vi "0926New Project.vi"() -> ()   [LabVIEW 2011] (continued)
                          }
                          frame #3 {
                            n542 = local read "Spec_midVar"() -> (w635:string)
                            n543 = property on="Cable AWG:" class="Ring (严格)"() -> ("StringsAndValues[]"=w648:T9)  [unwired: 2 in, 2 out]
                            n544 = property on="Customer" class="Ring (严格)"() -> ("StringsAndValues[]"=w650:T9)  [unwired: 2 in, 2 out]
                            n545 = Search and Replace String(replace all?=TRUE ("替换全部？(F)"), input string=w635, search string="#" ("搜索字符串"), replace string="\t") -> (result string=w639:string)  [unwired: 4 in, 3 out]
                            n546 = local read "Customer"() -> (w649:string)
                            n547 = local read "AWG"() -> (w647:string)
                            n548 = Spreadsheet String To Array(format string="%s" ("格式字符串"), spreadsheet string=w639, array type (2D Dbl)=string[][] []) -> (array=w642:string[][])  [unwired: 1 in]
                            n549 = call "_wmg_downlistValue.vi"(1:"Customer"=w647, 2:"Customer"=w648) -> ("Customer"=w651:u16)
                            n550 = call "_wmg_downlistValue.vi"(1:"Customer"=w649, 2:"Customer"=w650) -> ("Customer"=w652:u16)
                            n551 = Fract/Exp String To Number(string=w642) -> (number=w645:dbl[][])  [unwired: 3 in, 1 out]
                            n552 = local write "Cable AWG:"(w651) -> ()
                            n553 = local write "Customer"(w652) -> ()
                            n554 = local write "Spec _Data"(w645) -> ()
                            n555 = Array To Spreadsheet String(delimiter (Tab)="#" ("分隔符(Tab)"), array=w645, 3:"%s" ("格式字符串")) -> (spreadsheet string=w646:string)
                            n556 = local write "Spec String"(w646) -> ()
                          }
                        }
                      }
                    }
                  }
                  frame #1 {
                    # "列数\n0. S-para Pair Name\n1. NEXT Pair Name\n2. FEXT Pair Name\n3. Diff TestItems\n4. Single TestItems\n5. TDR TestItems\n6. Spec Associate\n7. VNA Cal File Path\n8. Report Config\n9. ILD Spec\n10. TDR Setting"
                    # "解析Prjinf"
                    n557 = local read "Project Information"() -> (w681:string)
                    n558 = Spreadsheet String To Array(delimiter (Tab)="#" ("分隔符(Tab)"), format string="%s" ("格式字符串"), spreadsheet string=w681, array type (2D Dbl)=string[][] []) -> (array=w678:string[][])
                    n559 = Index Array(array=w678, index (col) #1=0 ("索引"), index (col) #2=1 ("索引 (列)"), index (col) #3=2 ("索引 (列)"), index (col) #4=3 ("索引 (列)"), index (col) #5=4 ("索引 (列)"), index (col) #6=5 ("索引"), index (col) #7=6 ("索引 (列)"), index (col) #8=7 ("索引 (列)"), index (col) #9=8 ("索引 (列)"), index (col) #10=9 ("索引 (列)"), index (col) #11=10 ("索引"), index (col) #12=11 ("索引 (列)")) -> (element #1=w677:string[], element #2=w676:string[], element #3=w675:string[], element #4=w674:string[], element #5=w673:string[], element #6=w672:string[], element #7=w671:string[], element #8=w670:string[], element #9=w669:string[], element #10=w668:string[], element #11=w667:string[], element #12=w653:string[])  [unwired: 12 in]
                    n560 = stacked-sequence {
                      tunnel: w677 -> [_ w693 _ _ _]
                      tunnel: w676 -> [_ w692 _ _ _]
                      tunnel: w675 -> [_ w691 _ _ _]
                      tunnel: w674 -> [_ w690 _ _ _]
                      tunnel: w673 -> [_ w689 _ _ _]
                      tunnel: w672 -> [_ w688 _ _ _]
                      tunnel: w671 -> [_ _ w744 _ _]
                      tunnel: w670 -> [_ _ w743 _ _]
                      tunnel: w669 -> [_ _ _ w767 _]
                      tunnel: w668 -> [_ _ _ _ _]
                      tunnel: w667 -> [_ _ _ _ w785]
                      tunnel: w653 -> [_ _ w740 _ _]
                      frame #0 {
                        n561 = local read "Single init"() -> (→"Single init 2":i32[])
                        n562 = local read "NEXT init"() -> (→"NEXT init 2":i32[])
                        n563 = local read "FEXT init"() -> (→"FEXT init 2":i32[])
                        n564 = local read "S-p init"() -> (→"S-p init 2":i32[])
                        n565 = local read "Diff init"() -> (→"Diff init 2":i32[])
                        n566 = local read "TDR init"() -> (→"TDR init 2":i32[])
                      }
                      frame #1 {
                        n567 = stacked-sequence {
                          tunnel: [_ w715 _ _] -> _
                          tunnel: w693 -> [_ w715 _ _]
                          tunnel: w692 -> [_ w708 _ _]
                          tunnel: w691 -> [_ _ w721 _]
                          tunnel: w690 -> [_ _ w716 _]
                          tunnel: w689 -> [_ _ _ w729]
                          tunnel: w688 -> [_ _ _ w726]
                          frame #0 {
                            n568 = local read "FEXT init"() -> (w701:string[])
                            n569 = local read "FEXT init"() -> (w700:i32[])
                            n570 = local read "NEXT init"() -> (w704:string[])
                            n571 = local read "NEXT init"() -> (w702:i32[])
                            n572 = local read "S-p init"() -> (w703:i32[])
                            n573 = local read "S-p init"() -> (w705:string[])
                            n574 = property on="S-para Pair Name" class="LstBox (严格)"("Item Names"=w705, "Item Symbols"=w703) -> ()  [unwired: 2 in, 2 out]
                            n575 = property on="NEXT Pair Name" class="LstBox (严格)"("Item Names"=w704, "Item Symbols"=w702) -> ()  [unwired: 2 in, 2 out]
                            n576 = property on="FEXT Pair Name" class="LstBox (严格)"("Item Names"=w701, "Item Symbols"=w700) -> ()  [unwired: 2 in, 2 out]
                            n577 = local read "Single init"() -> (w697:string[])
                            n578 = local read "Single init"() -> (w696:i32[])
                            n579 = local read "TDR init"() -> (w695:string[])
                            n580 = local read "TDR init"() -> (w694:i32[])
                            n581 = local read "Diff init"() -> (w699:string[])
                            n582 = local read "Diff init"() -> (w698:i32[])
                            n583 = property on="Diff Test Items" class="LstBox (严格)"("Item Names"=w699, "Item Symbols"=w698) -> ()  [unwired: 2 in, 2 out]
                            n584 = property on="Single Test Items" class="LstBox (严格)"("Item Names"=w697, "Item Symbols"=w696) -> ()  [unwired: 2 in, 2 out]
                            n585 = property on="TDR Test Items" class="LstBox (严格)"("Item Names"=w695, "Item Symbols"=w694) -> ()  [unwired: 2 in, 2 out]
                          }
                          frame #1 {
                            n586 = local read "S-p init"() -> (w713:i32[])
                            n587 = local read "NEXT init"() -> (w706:string[])
                            n588 = local read "NEXT init"() -> (w709:i32[])
                            n589 = local read "S-p init"() -> (w707:string[])
                            n590 = call "_wmg_readItems.vi"("input_p"=w713, "input"=w707, "input_sp"=w715) -> ("output_p"=w712:i32[], "output_sp"=w714:string[])
                            n591 = call "_wmg_readItems2.vi"("input_p"=w709, "input"=w706, "input_sp"=w708) -> ("output_p"=w710:i32[], "output_sp"=w711:string[])
                            n592 = property on="S-para Pair Name" class="LstBox (严格)"("Item Names"=w714, "Item Symbols"=w712) -> ()  [unwired: 2 in, 2 out]
                            n593 = property on="NEXT Pair Name" class="LstBox (严格)"("Item Names"=w711, "Item Symbols"=w710) -> ()  [unwired: 2 in, 2 out]
                          }
                          frame #2 {
                            n594 = local read "FEXT init"() -> (w724:string[])
                            n595 = local read "FEXT init"() -> (w725:i32[])
                            n596 = local read "Diff init"() -> (w720:string[])
                            n597 = local read "Diff init"() -> (w719:i32[])
                            n598 = call "_wmg_readItems2.vi"("input_p"=w719, "input"=w720, "input_sp"=w716) -> ("output_p"=w718:i32[], "output_sp"=w717:string[])
                            n599 = call "_wmg_readItems.vi"("input_p"=w725, "input"=w724, "input_sp"=w721) -> ("output_p"=w722:i32[], "output_sp"=w723:string[])
                            n600 = property on="FEXT Pair Name" class="LstBox (严格)"("Item Names"=w723, "Item Symbols"=w722) -> ()  [unwired: 2 in, 2 out]
                            n601 = property on="Diff Test Items" class="LstBox (严格)"("Item Names"=w717, "Item Symbols"=w718) -> ()  [unwired: 2 in, 2 out]
                          }
                          frame #3 {
                            n602 = local read "TDR init"() -> (w728:string[])
                            n603 = local read "TDR init"() -> (w727:i32[])
                            n604 = local read "Single init"() -> (w730:string[])
                            n605 = local read "Single init"() -> (w731:i32[])
                            n606 = call "_wmg_readItems.vi"("input_p"=w731, "input"=w730, "input_sp"=w729) -> ("output_p"=w733:i32[], "output_sp"=w732:string[])
                            n607 = call "_wmg_readItems2.vi"("input_p"=w727, "input"=w728, "input_sp"=w726) -> ("output_p"=w735:i32[], "output_sp"=w734:string[])
                            n608 = property on="TDR Test Items" class="LstBox (严格)"("Item Names"=w734, "Item Symbols"=w735) -> ()  [unwired: 2 in, 2 out]
                            n609 = property on="Single Test Items" class="LstBox (严格)"("Item Names"=w732, "Item Symbols"=w733) -> ()  [unwired: 2 in, 2 out]
                          }
                        }
                      }
                      frame #2 {
                        n610 = property on="Diff Test Items" class="LstBox (严格)"() -> ("Item Symbols"=w749:i32[], "Item Names"=w747:string[])  [unwired: 2 in, 2 out]
                        n611 = Index Array(array=w743, index=0 ("索引")) -> (element=w742:string)
                        n612 = Index Array(array=w740, index=0 ("索引")) -> (element=w738:string)
                        n613 = local write "VNA Cal File Path:"(w742) -> ()
                        n614 = Equal?(x=w738, y="TRUE") -> (x = y?=w736:bool)
                        n615 = for {
                          tunnel: w749 -> [w755] mode=indexing
                          shift-right: [w750] -> w746
                          shift-left: string[] [] -> [w751]
                          tunnel: w747 -> [w752] mode=indexing
                          n616 = Equal?(x=w755, y=38) -> (x = y?=w753:bool)
                          n617 = case shown="假" w753 {
                            tunnel: w752 -> [_ w759]
                            tunnel: w751 -> [w756 w758]
                            tunnel: [w756 w757] -> w750
                            frame False {
                            }
                            frame True {
                              n618 = Insert Into Array(array=w758, new element=w759) -> (w757:string[])  [unwired: 1 in]
                            }
                          }
                        }
                        n619 = local write "cancel dem2X?"(w736) -> ()
                        n620 = Build Array(w746, w744) -> (w745:string[][])
                        n621 = local write "Spec Associate"(w745) -> ()
                      }
                      frame #3 {
                        n622 = Index Array(array=w767, index #1=0 ("索引"), index #3=2 ("索引")) -> (element #1=w764:string, element #2=w763:string, element #3=w761:string)  [unwired: 1 in]
                        n623 = String To Path(string=w764) -> (path=w765:path)
                        n624 = call "_wmg_ReportConfigDivided@.vi"("Input"=w763) -> ("Output"=w762:string[][])
                        n625 = call "_wmg_ReportConfigDivided@.vi"("Input"=w761) -> ("Output"=w760:string[][])
                        n626 = local write "Postion for Raw data"(w762) -> ()
                        n627 = local write "Report Templete Path:"(w765) -> ()
                        n628 = local write "Postion for \"PN&Tester&Date\" etc Fields"(w760) -> ()
                      }
                      frame #4 {
                        # "TDR Setting\n0. Start TimeNs\n1. Stop TimeNs\n2. Data Points\n3. Filter Risetime(ps)\n4. Compensation(ohm)\n5. Impedance Filter\n6. Impedance Spec:\n7. Delay Spec:\n8. skew Spec:\n9. IL 2X Data:"
                        n629 = Index Array(array=w785, index #1=0 ("索引"), index #2=1 ("索引"), index #3=2 ("索引"), index #4=3 ("索引"), index #5=4 ("索引"), index #6=5 ("索引"), index #7=6 ("索引"), index #8=9 ("索引")) -> (element #1=w777:string, element #2=w776:string, element #3=w775:string, element #4=w774:string, element #5=w773:string, element #6=w772:string, element #7=w771:string, element #8=w769:string)
                        n630 = stacked-sequence {
                          tunnel: w777 -> [w810]
                          tunnel: w776 -> [w807]
                          tunnel: w775 -> [w805]
                          tunnel: w774 -> [w804]
                          tunnel: w773 -> [w801]
                          tunnel: w772 -> [w799]
                          tunnel: w771 -> [w796]
                          tunnel: w769 -> [w791]
                          frame #0 {
                            n631 = call "_wmg_ImpSpecDivided@.vi"("Input"=w796) -> ("Output"=w795:string[][])
                            n632 = Spreadsheet String To Array(format string="%s" ("格式字符串"), spreadsheet string=w791, array type (2D Dbl)=dbl[] []) -> (array=w786:dbl[])  [unwired: 1 in]
                            n633 = Insert Into Array(array=w795, index (col)=0 ("禁用的索引 (列)"), new element=string[] ["Mating Area", "Cable Area"]) -> (w793:string[][])  [unwired: 1 in]
                            n634 = local write "2X Thru  IL Data"(w786) -> ()
                            n635 = Decimal String To Number(string=w799) -> (offset past number=w800:i32)  [unwired: 2 in, 1 out]
                            n636 = local write "Impedance Spec:"(w793) -> ()
                            n637 = Number To Boolean Array(number=w800) -> (Boolean array=w798:bool[])
                            n638 = Array To Spreadsheet String(array=w786, 3:"%s" ("格式字符串")) -> (spreadsheet string=w788:string)  [unwired: 1 in]
                            n639 = Fract/Exp String To Number(string=w801) -> (number=w802:dbl)  [unwired: 3 in, 1 out]
                            n640 = Index Array(array=w798) -> (element=w797:bool)  [unwired: 1 in]
                            n641 = Fract/Exp String To Number(string=w807) -> (number=w808:dbl)  [unwired: 3 in, 1 out]
                            n642 = Decimal String To Number(string=w805) -> (number=w806:i32)  [unwired: 2 in, 1 out]
                            n643 = Fract/Exp String To Number(string=w804) -> (number=w803:dbl)  [unwired: 3 in, 1 out]
                            n644 = local write "2X Thru String"(w788) -> ()
                            n645 = local write "Compensation(ohm)"(w802) -> ()
                            n646 = Fract/Exp String To Number(string=w810) -> (number=w809:dbl)  [unwired: 3 in, 1 out]
                            n647 = local write "Filter Risetime(ps)"(w803) -> ()
                            n648 = local write "Impedance Filter"(w797) -> ()
                            n649 = local write "Start TimeNs"(w809) -> ()
                            n650 = local write "StopTimeNs"(w808) -> ()
                            n651 = local write "Data Points"(w806) -> ()
                          }
                        }
                      }
                    }
                  }
                  frame #2 {
                    w819 = T3 {"Row"=0, "Column"=0} ("编辑位置")
                    w820 = u32 4 ("列数")
                    n652 = property on="Single Test Items" class="LstBox (严格)"() -> ("Item Names"=w827:string[], "Item Symbols"=w826:i32[])  [unwired: 2 in, 2 out]
                    n653 = property on="TDR Test Items" class="LstBox (严格)"() -> ("Item Names"=w825:string[], "Item Symbols"=w824:i32[])  [unwired: 2 in, 2 out]
                    n654 = property on="Diff Test Items" class="LstBox (严格)"() -> ("Item Names"=w829:string[], "Item Symbols"=w828:i32[])  [unwired: 2 in, 2 out]
                    n655 = call "_wmg_SelectItems2.vi"("Item Syms"=w824, "Item name"=w825) -> ("Selected tem"=w823:string[])  [unwired: 7 in, 2 out]
                    n656 = call "_wmg_SelectItems2.vi"("Item Syms"=w828, "Item name"=w829) -> ("Selected tem"=w822:string[])  [unwired: 7 in, 2 out]
                    n657 = call "_wmg_SelectItems2.vi"("Item Syms"=w826, "Item name"=w827) -> ("Selected tem"=w821:string[])  [unwired: 7 in, 2 out]
                    n658 = property on="Postion for Raw data" class="Tbl (严格)"() -> ("Value"=w818:string[][])  [unwired: 2 in, 2 out]
                    n659 = Insert Into Array(array=w823, new element #1=w822, new element #2=w821) -> (w817:string[])  [unwired: 1 in]
                    n660 = local read "2X Thru  IL Data"() -> (w813:dbl[])
                    n661 = Replace Array Subset(array=w818, new element=w817, index (col)=0 ("禁用的索引 (列)")) -> (w816:string[][])  [unwired: 1 in]
                    n662 = property on="Postion for Raw data" class="Tbl (严格)"("Value"=w816) -> ()  [unwired: 2 in, 2 out]
                    n663 = Array Size(array=w813) -> (size(s)=w812:i32)
                    n664 = for {
                      N: w812 -> [_]
                      tunnel: [w830] -> w811 mode=indexing
                      i -> [w830]
                    }
                    n665 = Bundle(w811, "2X Thru  IL Data"=w813) -> (w814:cluster{i32[], "2X Thru  IL Data":dbl[]})  [unwired: 1 in]
                    n666 = local write "Insertion Loss"(w814) -> ()
                    n667 = property on="Postion for Raw data" class="Tbl (严格)"("Number of Columns"=w820, "EditPos"=w819) -> ()  [unwired: 2 in, 2 out]
                    n668 = property on="Postion for \"PN&Tester&Date\" etc Fields" class="Tbl (严格)"("Number of Columns"=w820, "EditPos"=w819) -> ()  [unwired: 2 in, 2 out]
                  }
                  frame #3 {
                    n669 = local read "Local"() -> (w831:bool)
                    n670 = case shown="真" w831 {
                      frame False {
                        n671 = local read "result_query"() -> (w835:string)
                        n672 = call <vilib>:"Trim Whitespace.vi"("string"=w835) -> ("trimmed string"=w834:string)  [unwired: 1 in]
                        n673 = String Length(string=w834) -> (length=w833:i32)
                        n674 = Equal To 0?(x=w833) -> (x = 0?=w832:bool)
                        n675 = case shown="假" w832 {
                          frame False {
                            n676 = property on="Update" class="Bool (严格)"("DisabledEnum"=T4."Enabled" ("禁用")) -> ()  [unwired: 2 in, 2 out]
                            n677 = property on="Delete" class="Bool (严格)"("DisabledEnum"=T4."Enabled" ("禁用")) -> ()  [unwired: 2 in, 2 out]
                          }
                          frame True {
                            n678 = local write "Luxshare_P/N:"("") -> ()
                            n679 = One Button Dialog(message="数据库中无此记录" ("消息")) -> ()  [unwired: 1 in, 1 out]
                          }
                        }
                      }
                      frame True {
                        n680 = local read "fileexist"() -> (w841:bool)
                        n681 = Not(x=w841) -> (.not. x?=w840:bool)
                        n682 = case shown="真" w840 {
                          frame False {
                            # "文件不存在"
                            n683 = local read "Impedance Spec:"() -> (w845:string[][])
                            n684 = local write "Luxshare_P/N:"("") -> ()
                            n685 = Replace Array Subset(array=w845, new element=string[] ["", "", ""] ("新元素/子数组"), index (col)=0 ("禁用的索引 (列)")) -> (w844:string[][])  [unwired: 1 in]
                            n686 = local write "Impedance Spec:"(w844) -> ()
                            n687 = property on="Update" class="Bool (严格)"("DisabledEnum"=T4."Disabled and Grayed Out" ("禁用")) -> ()  [unwired: 2 in, 2 out]
                            n688 = property on="Delete" class="Bool (严格)"("DisabledEnum"=T4."Disabled and Grayed Out" ("禁用")) -> ()  [unwired: 2 in, 2 out]
                          }
                          frame True {
                            n689 = property on="Update" class="Bool (严格)"("DisabledEnum"=T4."Enabled" ("禁用")) -> ()  [unwired: 2 in, 2 out]
                            n690 = property on="Delete" class="Bool (严格)"("DisabledEnum"=T4."Enabled" ("禁用")) -> ()  [unwired: 2 in, 2 out]
                          }
                        }
                      }
                    }
                  }
                }
              }
              frame 100 {
                n691 = stacked-sequence {
                  frame #0 {
                    n692 = local read "Local"() -> (w851:bool)
                    n693 = case shown="假" w851 {
                      frame False {
                        n694 = property on="System_Mode" class="Ring (严格)"() -> ("RingText.Text"=w854:string)  [unwired: 2 in, 2 out]
                        n695 = local read "Luxshare_P/N:"() -> (w856:string)
                        n696 = call "_wmg_HardModetoHardModewhereConnect.vi"("Input"=w854) -> ("Output"=w855:string)
                        n697 = call "_wmg_PNtoPNwhereConnect.vi"("Input"=w856) -> ("Output"=w853:string)
                        n698 = Concatenate Strings(w853, w855) -> (w852:string)
                        n699 = call "sql-delete.vi"("操作模式"=T8."删除数据", "限定条件"=w852) -> ()  [unwired: 16 in, 2 out]
                      }
                      frame True {
                        n700 = local read "Luxshare_P/N:"() -> (w859:string)
                        n701 = call <vilib>:"Application Directory.vi"() -> ("Application Directory"=w863:path)
                        n702 = Concatenate Strings("Database\\" ("字符串"), w859, ".hpj" ("字符串")) -> (w862:string)
                        n703 = Build Path(base path=w863, name or relative path=w862) -> (appended path=w858:path)
                        n704 = Delete(path (use dialog)=w858) -> ()  [unwired: 4 in, 3 out]
                      }
                    }
                  }
                  frame #1 {
                    n705 = stacked-sequence {
                      frame #0 {
                        w878 = "@"
                        w879 = "\r\n"
                        w888 = "%s" ("格式字符串")
                        n706 = local read "Impedance Filter"() -> (w865:bool)
                        n707 = local read "Impedance Spec:"() -> (w890:string[][])
                        n708 = local read "2X Thru String"() -> (w875:string)
                        n709 = property on="Skew max(ps)" class="DigNum (严格)"() -> ("NumText.Text"=w867:string)  [unwired: 2 in, 2 out]
                        n710 = property on="Delay(ns)" class="DigNum (严格)"() -> ("NumText.Text"=w874:string)  [unwired: 2 in, 2 out]
                        n711 = property on="Start TimeNs" class="DigNum (严格)"() -> ("NumText.Text"=w873:string)  [unwired: 2 in, 2 out]
                        n712 = property on="StopTimeNs" class="DigNum (严格)"() -> ("NumText.Text"=w872:string)  [unwired: 2 in, 2 out]
                        n713 = property on="Data Points" class="DigNum (严格)"() -> ("NumText.Text"=w871:string)  [unwired: 2 in, 2 out]
                        n714 = property on="Filter Risetime(ps)" class="DigNum (严格)"() -> ("NumText.Text"=w870:string)  [unwired: 2 in, 2 out]
                        n715 = property on="Compensation(ohm)" class="DigNum (严格)"() -> ("NumText.Text"=w869:string)  [unwired: 2 in, 2 out]
                        n716 = Boolean To (0,1)(Boolean=w865) -> (0, 1=w892:i16)
                        n717 = Number To Decimal String(number=w892) -> (decimal integer string=w891:string)  [unwired: 1 in]
                        n718 = call "impedance spec.vi"("Impedance Spec:"=w890) -> ("Impedance spec string"=w889:string)  [unwired: 10 in]
                        n719 = call <vilib>:"Trim Whitespace.vi"("string"=w875) -> ("trimmed string"=w864:string)  [unwired: 1 in]
                        n720 = Build Array(w873, w872, w871, w870, w869, w891, w889, w874, w867, w864) -> (w868:string[])
                        n721 = local read "Report Templete Path:"() -> (w876:path)
                        n722 = property on="Postion for Raw data" class="Tbl (严格)"() -> ("Value"=w887:string[][])  [unwired: 2 in, 2 out]
                        n723 = local write "TDR Setting"(w868) -> ()
                        n724 = property on="Postion for \"PN&Tester&Date\" etc Fields" class="Tbl (严格)"() -> ("Value"=w886:string[][])  [unwired: 2 in, 2 out]
                        n725 = Array To Spreadsheet String(array=w887, 3:w888) -> (spreadsheet string=w884:string)  [unwired: 1 in]
                        n726 = Array To Spreadsheet String(array=w886, 3:w888) -> (spreadsheet string=w882:string)  [unwired: 1 in]
                        n727 = Path To String(path=w876) -> (string=w877:string)
                        n728 = Search and Replace String(replace all?=TRUE ("替换全部？(F)"), input string=w884, search string=w879, replace string=w878) -> (result string=w881:string)  [unwired: 4 in, 3 out]
                        n729 = Search and Replace String(replace all?=TRUE ("替换全部？(F)"), input string=w882, search string=w879, replace string=w878) -> (result string=w880:string)  [unwired: 4 in, 3 out]
                        n730 = Build Array(w877, w881, w880) -> (w866:string[])
                        n731 = local write "Report Config"(w866) -> ()
                      }
                      frame #1 {
                        n732 = property on="S-para Pair Name" class="LstBox (严格)"() -> ("Item Names"=w926:string[], "Item Symbols"=w925:i32[])  [unwired: 2 in, 2 out]
                        n733 = property on="NEXT Pair Name" class="LstBox (严格)"() -> ("Item Names"=w924:string[], "Item Symbols"=w923:i32[])  [unwired: 2 in, 2 out]
                        n734 = property on="FEXT Pair Name" class="LstBox (严格)"() -> ("Item Names"=w922:string[], "Item Symbols"=w921:i32[])  [unwired: 2 in, 2 out]
                        n735 = local read "Spec Associate"() -> (w915:string[][])
                        n736 = property on="Single Test Items" class="LstBox (严格)"() -> ("Item Names"=w928:string[], "Item Symbols"=w927:i32[])  [unwired: 2 in, 2 out]
                        n737 = property on="Diff Test Items" class="LstBox (严格)"() -> ("Item Names"=w930:string[], "Item Symbols"=w929:i32[])  [unwired: 2 in, 2 out]
                        n738 = property on="TDR Test Items" class="LstBox (严格)"() -> ("Item Names"=w906:string[], "Item Symbols"=w905:i32[])  [unwired: 2 in, 2 out]
                        n739 = call "Selected items.vi"("Item Syms"=w925, "Item name"=w926) -> ("Selected tem"=w920:string[])  [unwired: 7 in, 2 out]
                        n740 = call "Selected items.vi"("Item Syms"=w923, "Item name"=w924) -> ("Selected tem"=w919:string[])  [unwired: 7 in, 2 out]
                        n741 = call "Selected items.vi"("Item Syms"=w921, "Item name"=w922) -> ("Selected tem"=w918:string[])  [unwired: 7 in, 2 out]
                        n742 = call "Selected items.vi"("Item Syms"=w929, "Item name"=w930) -> ("Selected tem"=w917:string[])  [unwired: 7 in, 2 out]
                        n743 = call "Selected items.vi"("Item Syms"=w927, "Item name"=w928) -> ("Selected tem"=w916:string[])  [unwired: 7 in, 2 out]
                        n744 = call "Selected items.vi"("Item Syms"=w905, "Item name"=w906) -> ("Selected tem"=w903:string[])  [unwired: 7 in, 2 out]
                        n745 = Index Array(array=w915, index (row)=1 ("索引 (行)")) -> (element=w904:string[])  [unwired: 1 in]
                        n746 = local read "VNA Cal File Path:"() -> (w900:string)
                        n747 = local read "cancel dem2X?"() -> (w896:bool)
                        n748 = local read "ILD Spec"() -> (w899:u16)
                        n749 = local read "Report Config"() -> (w901:string[])
                        n750 = local read "TDR Setting"() -> (w902:string[])
                        n751 = Number To Decimal String(number=w899) -> (decimal integer string=w908:string)  [unwired: 1 in]
                        n752 = Build Array(w900) -> (w913:string[])
                        n753 = Select(t="TRUE", s=w896, f="FALSE") -> (s? t:f=w893:string)
                        n754 = Build Array(w908) -> (w907:string[])
                        n755 = Build Array(w893) -> (w897:string[])
                        n756 = Build Array(w920, w919, w918, w917, w916, w903, w904, w913, w901, w907, w902, w897) -> (w912:string[][])
                        n757 = Transpose 2D Array(2D array=w912) -> (transposed array=w911:string[][])
                        n758 = Array To Spreadsheet String(delimiter (Tab)="#" ("分隔符(Tab)"), array=w911, 3:"%s" ("格式字符串")) -> (spreadsheet string=w898:string)
                        n759 = local write "Project Information"(w898) -> ()
                      }
                      frame #2 {
                        n760 = local read "VNA Cal File Path:"() -> (w950:string)
                        n761 = property on="Diff Test Items" class="LstBox (严格)"() -> ("Item Symbols"=w947:i32[])  [unwired: 2 in, 2 out]
                        n762 = property on="Single Test Items" class="LstBox (严格)"() -> ("Item Symbols"=w946:i32[])  [unwired: 2 in, 2 out]
                        n763 = property on="TDR Test Items" class="LstBox (严格)"() -> ("Item Symbols"=w945:i32[])  [unwired: 2 in, 2 out]
                        n764 = property on="S-para Pair Name" class="LstBox (严格)"() -> ("Item Symbols"=w944:i32[])  [unwired: 2 in, 2 out]
                        n765 = property on="NEXT Pair Name" class="LstBox (严格)"() -> ("Item Symbols"=w943:i32[])  [unwired: 2 in, 2 out]
                        n766 = property on="FEXT Pair Name" class="LstBox (严格)"() -> ("Item Symbols"=w939:i32[])  [unwired: 2 in, 2 out]
                        n767 = local read "Luxshare_P/N:"() -> (w937:string)
                        n768 = local read "Length(mm):"() -> (w951:string)
                        n769 = String Length(string=w937) -> (length=w938:i32)
                        n770 = Empty String/Path?(string/path=w950) -> (empty?=w948:bool)
                        n771 = Empty String/Path?(string/path=w951) -> (empty?=w949:bool)
                        n772 = Build Array(w947, w946, w945, w944, w943, w939) -> (w942:i32[][])
                        n773 = Not(x=w949) -> (.not. x?=w941:bool)
                        n774 = Not(x=w948) -> (.not. x?=w940:bool)
                        n775 = Greater Than 0?(x=w938) -> (x > 0?=w936:bool)
                        n776 = call "_wmg_whetherItemsEmpty.vi"("Input"=w942) -> ("bool"=w952:bool)
                        n777 = Compound Arithmetic op=AND(w936, w941, w940, w952) -> (w935:bool)
                        n778 = local write "save?"(w935) -> ()
                        n779 = local read "Spec _Data"() -> (w933:dbl[][])
                        n780 = Array To Spreadsheet String(delimiter (Tab)="#" ("分隔符(Tab)"), array=w933, 3:"%s" ("格式字符串")) -> (spreadsheet string=w934:string)
                        n781 = local write "Spec String"(w934) -> ()
                      }
                      frame #3 {
                        n782 = local read "Local"() -> (w953:bool)
                        n783 = case shown="真" w953 {
                          frame False {
                            # "17"
                            # "16"
                            # "15"
                            # "14"
                            # "13"
                            # "11"
                            # "10"
                            # "9"
                            # "8"
                            # "7"
                            # "6"
                            # "5"
                            # "4"
                            # "3"
                            # "2"
                            # "1"
                            n784 = local read "Label Print?"() -> (w959:bool)
                            n785 = local read "fre-save"() -> (w966:string[])
                            n786 = Boolean To (0,1)(Boolean=w959) -> (0, 1=w984:i16)
                            n787 = local read "EEPROM Write/Read ?"() -> (w960:bool)
                            n788 = local read "Sample Description:"() -> (w980:string)
                            n789 = local read "Project Information"() -> (w981:string)
                            n790 = Array To Spreadsheet String(delimiter (Tab)="," ("分隔符(Tab)"), array=w966, 3:"" ("格式字符串")) -> (spreadsheet string=w963:string)
                            n791 = Number To Decimal String(number=w984) -> (decimal integer string=w974:string)  [unwired: 1 in]
                            n792 = local read "Customer_P/N:"() -> (w983:string)
                            n793 = local read "Switch File Path"() -> (w958:string)
                            n794 = local read "Switch Matrix"() -> (w976:string)
                            n795 = local read "Label Content"() -> (w973:string)
                            n796 = local read "Length(mm):"() -> (w978:string)
                            n797 = local read "Spec String"() -> (w977:string)
                            n798 = call <vilib>:"Trim Whitespace.vi"("string"=w963) -> ("trimmed string"=w962:string)  [unwired: 1 in]
                            n799 = property on="Customer" class="Ring (严格)"() -> ("RingText.Text"=w982:string)  [unwired: 2 in, 2 out]
                            n800 = property on="Cable AWG:" class="Ring (严格)"() -> ("RingText.Text"=w979:string)  [unwired: 2 in, 2 out]
                            n801 = local read "FixtureNo"() -> (w971:string)
                            n802 = local read "Label Num"() -> (w986:string)
                            n803 = local read "Remark:"() -> (w972:string)
                            n804 = Boolean To (0,1)(Boolean=w960) -> (0, 1=w985:i16)
                            n805 = local read "AutoSN"() -> (w968:bool)
                            n806 = Number To Decimal String(number=w985) -> (decimal integer string=w975:string)  [unwired: 1 in]
                            n807 = Boolean To (0,1)(Boolean=w968) -> (0, 1=w969:i16)
                            n808 = Number To Decimal String(number=w969) -> (decimal integer string=w967:string)  [unwired: 1 in]
                            n809 = local read "Luxshare_P/N:"() -> (w970:string)
                            n810 = local read "Spec File Path"() -> (w957:string)
                            n811 = local read "Spec Points"() -> (w956:dbl)
                            n812 = property on="System_Mode" class="Ring (严格)"() -> ("RingText.Text"=w954:string)  [unwired: 2 in, 2 out]
                            n813 = Number To Decimal String(number=w956) -> (decimal integer string=w955:string)  [unwired: 1 in]
                            n814 = Build Array(w970, w983, w982, w981, w980, w979, w978, w977, w976, w975, w971, w974, w986, w973, w972, w967, w962, w958, w957, w955, w954) -> (w961:string[])
                            n815 = local write "Project File"(w961) -> ()
                          }
                          frame True {
                            # "20"
                            # "19"
                            # "11"
                            # "10"
                            # "9"
                            # "8"
                            # "7"
                            # "6"
                            # "5"
                            # "4"
                            # "3"
                            # "2"
                            # "1"
                            n816 = local read "Label Print?"() -> (w993:bool)
                            n817 = local read "fre-save"() -> (w1000:string[])
                            n818 = Boolean To (0,1)(Boolean=w993) -> (0, 1=w1018:i16)
                            n819 = local read "EEPROM Write/Read ?"() -> (w995:bool)
                            n820 = local read "Sample Description:"() -> (w1014:string)
                            n821 = local read "Project Information"() -> (w1015:string)
                            n822 = Array To Spreadsheet String(delimiter (Tab)="," ("分隔符(Tab)"), array=w1000, 3:"" ("格式字符串")) -> (spreadsheet string=w997:string)
                            n823 = local read "SNType"() -> (w994:string)
                            n824 = Number To Decimal String(number=w1018) -> (decimal integer string=w1008:string)  [unwired: 1 in]
                            n825 = local read "Customer_P/N:"() -> (w1017:string)
                            n826 = local read "Switch Matrix"() -> (w1010:string)
                            n827 = local read "Label Content"() -> (w1007:string)
                            n828 = local read "Length(mm):"() -> (w1012:string)
                            n829 = local read "Spec String"() -> (w1011:string)
                            n830 = property on="CmdType" class="Ring (严格)"() -> ("RingText.Text"=w992:string)  [unwired: 2 in, 2 out]
                            n831 = call <vilib>:"Trim Whitespace.vi"("string"=w997) -> ("trimmed string"=w989:string)  [unwired: 1 in]
                            n832 = property on="Customer" class="Ring (严格)"() -> ("RingText.Text"=w1016:string)  [unwired: 2 in, 2 out]
                            n833 = property on="Cable AWG:" class="Ring (严格)"() -> ("RingText.Text"=w1013:string)  [unwired: 2 in, 2 out]
                            n834 = local read "FixtureNo"() -> (w1005:string)
                            n835 = local read "Label Num"() -> (w1020:string)
                            n836 = local read "Remark:"() -> (w1006:string)
                            n837 = local read "Switch File Path"() -> (w990:string)
                            n838 = Boolean To (0,1)(Boolean=w995) -> (0, 1=w1019:i16)
                            n839 = local read "AutoSN"() -> (w1002:bool)
                            n840 = Number To Decimal String(number=w1019) -> (decimal integer string=w1009:string)  [unwired: 1 in]
                            n841 = Boolean To (0,1)(Boolean=w1002) -> (0, 1=w1003:i16)
                            n842 = Number To Decimal String(number=w1003) -> (decimal integer string=w1001:string)  [unwired: 1 in]
                            n843 = local read "Luxshare_P/N:"() -> (w1004:string)
                            n844 = local read "Spec File Path"() -> (w991:string)
                            n845 = local read "Spec Points"() -> (w988:dbl)
                            n846 = Number To Decimal String(number=w988) -> (decimal integer string=w987:string)  [unwired: 1 in]
                            n847 = Build Array(w1004, w1017, w1016, w1015, w1014, w1013, w1012, w1011, w1010, w1009, w992, w994, w1005, w1008, w1020, w1007, w1006, w1001, w989, w990, w991, w987) -> (w996:string[])
                            n848 = local write "Project File"(w996) -> ()
                          }
                        }
                      }
                      frame #4 {
                        n849 = local read "save?"() -> (w1021:bool)
                        n850 = case shown="真" w1021 {
                          frame False {
                            n851 = One Button Dialog(message="保存信息不完整" ("消息")) -> ()  [unwired: 1 in, 1 out]
                          }
                          frame True {
                            n852 = local read "Luxshare_P/N:"() -> (w1025:string)
                            n853 = local read "Project File"() -> (w1024:string[])
                            n854 = local read "Local"() -> (w1023:bool)
                            n855 = case shown="假" w1023 {
                              tunnel: w1024 -> [w1029 w1041]
                              tunnel: w1025 -> [_ w1049]
                              frame False {
                                (unwired) string[] ["LuxsharePN", "CustomerPN", "Customer", "Prjinf", "SampleDes", "AWG", "Length", "Spec", "SwitchMatrix", "EEPROMTF", "FixtureNo", "LabelTF", "LabelNum", "LabelC", "Remark", "AutoSN", "FrePoints"] ("列名")
                                # "保存至数据库"
                                n856 = call "sql-writeinfo_vproject.vi"("操作模式"=enum16{"写入数据", "更改数据"}."写入数据", "列名"=string[] ["LuxsharePN", "CustomerPN", "Customer", "Prjinf", "SampleDes", "AWG", "Length", "Spec", "SwitchMatrix", "EEPROMTF", "FixtureNo", "LabelTF", "LabelNum", "LabelC", "Remark", "AutoSN", "FrePoints", "Switch_File_Path", "Spec_File_Path", "Spec_Points", "HardWare_Mode"], "值"=w1029) -> ("简单报错"=w1027:string, "status"=w1028:bool)  [unwired: 15 in]
                                n857 = case shown="真" w1028 {
                                tunnel: w1027 -> [_ w1040]
                                frame False {
                                # "清空操作"
                                n858 = control-ref of="Report Templete Path:"() -> (w1034:refnum<vi>)
                                n859 = control-ref of="Data Points"() -> (w1033:refnum<vi>)
                                n860 = control-ref of="Spec _Data"() -> (w1032:refnum<vi>)
                                n861 = local read "bool"() -> (w1031:refnum<vi>[])
                                n862 = One Button Dialog(message="Save Finished!" ("消息")) -> ()  [unwired: 1 in, 1 out]
                                n863 = local read "number"() -> (w1035:refnum<vi>[])
                                n864 = local read "string"() -> (w1038:refnum<vi>[])
                                n865 = local read "chart"() -> (w1036:refnum<vi>[])
                                n866 = local read "list"() -> (w1037:refnum<vi>[])
                                n867 = call "_wmg_initAllCtrls.vi"("chart"=w1036, "number"=w1035, "list"=w1037, "string"=w1038, "bool"=w1031, "Spec _Data"=w1032, "Data Points"=w1033, "Report Templete Path:"=w1034) -> ()
                                }
                                frame True {
                                n868 = One Button Dialog(message=w1040) -> ()  [unwired: 1 in, 1 out]
                                }
                                }
                              }
                              frame True {
                                n869 = call <vilib>:"Application Directory.vi"() -> ("Application Directory"=w1048:path)
                                n870 = Concatenate Strings("Database\\" ("字符串"), w1049, ".hpj" ("字符串")) -> (w1047:string)
                                n871 = Build Path(base path=w1048, name or relative path=w1047) -> (appended path=w1044:path)
                                n872 = call <vilib>:"Check if File or Folder Exists.vi"("path"=w1044) -> ("file or folder exists?"=w1043:bool, "dup path"=w1042:path)  [unwired: 8 in, 1 out]
                                n873 = case shown="假" w1043 {
                                tunnel: w1042 -> [w1052 w1063]
                                tunnel: w1041 -> [w1051 w1062]
                                frame False {
                                # "清空操作"
                                n874 = One Button Dialog(message="Local file save Finished!" ("消息")) -> ()  [unwired: 1 in, 1 out]
                                n875 = control-ref of="Report Templete Path:"() -> (w1058:refnum<vi>)
                                n876 = control-ref of="Data Points"() -> (w1059:refnum<vi>)
                                n877 = control-ref of="Spec _Data"() -> (w1060:refnum<vi>)
                                n878 = local read "bool"() -> (w1050:refnum<vi>[])
                                n879 = Write to Binary File(file (use dialog)=w1052, data=w1051, 9:T7."big-endian, network order" ("字节顺序(0:big-endian, network order)")) -> ()  [unwired: 3 in, 3 out]
                                n880 = local read "number"() -> (w1057:refnum<vi>[])
                                n881 = local read "string"() -> (w1054:refnum<vi>[])
                                n882 = local read "chart"() -> (w1056:refnum<vi>[])
                                n883 = local read "list"() -> (w1055:refnum<vi>[])
                                n884 = call "_wmg_initAllCtrls.vi"("chart"=w1056, "number"=w1057, "list"=w1055, "string"=w1054, "bool"=w1050, "Spec _Data"=w1060, "Data Points"=w1059, "Report Templete Path:"=w1058) -> ()
                                }
                                frame True {
                                n885 = Two Button Dialog(message="该PN的文件已经存在\n是否覆盖？", 1:"取消" ("F按钮名称（“取消”）"), 2:"覆盖" ("T按钮名称（“确定”）")) -> (T button?=w1064:bool)
                                n886 = case shown="真" w1064 {
                                tunnel: w1063 -> [_ w1069]
                                tunnel: w1062 -> [_ w1068]
                                frame False {
                                }
                                frame True {
                                n887 = stacked-sequence {
                                tunnel: w1069 -> [w1072 _]
                                tunnel: w1068 -> [w1070 _]
                                frame #0 {
                                n888 = One Button Dialog(message="Coved successfully!" ("消息")) -> ()  [unwired: 1 in, 1 out]
                                n889 = Write to Binary File(file (use dialog)=w1072, data=w1070, 9:T7."big-endian, network order" ("字节顺序(0:big-endian, network order)")) -> ()  [unwired: 3 in, 3 out]
                                }
                                frame #1 {
                                # "清空操作"
                                n890 = control-ref of="Report Templete Path:"() -> (w1078:refnum<vi>)
                                n891 = control-ref of="Data Points"() -> (w1079:refnum<vi>)
                                n892 = control-ref of="Spec _Data"() -> (w1080:refnum<vi>)
                                n893 = local read "number"() -> (w1077:refnum<vi>[])
                                n894 = local read "string"() -> (w1074:refnum<vi>[])
                                n895 = local read "chart"() -> (w1076:refnum<vi>[])
                                n896 = local read "list"() -> (w1075:refnum<vi>[])
                                n897 = call "_wmg_initAllCtrls.vi"("chart"=w1076, "number"=w1077, "list"=w1075, "string"=w1074, "Spec _Data"=w1080, "Data Points"=w1079, "Report Templete Path:"=w1078) -> ()  [unwired: 1 in]
                                }
                                }
                                }
                                }
                                }
                                }
                              }
                            }
                          }
                        }
                      }
                      frame #5 {
                        n898 = property on="Update" class="Bool (严格)"("DisabledEnum"=T4."Disabled and Grayed Out" ("禁用")) -> ()  [unwired: 2 in, 2 out]
                        n899 = property on="Delete" class="Bool (严格)"("DisabledEnum"=T4."Disabled and Grayed Out" ("禁用")) -> ()  [unwired: 2 in, 2 out]
                        n900 = property on="Luxshare_P/N:" class="Str"("DisabledEnum"=T4."Disabled and Grayed Out" ("禁用")) -> ()  [unwired: 2 in, 2 out]
                        n901 = local write "Query"(FALSE ("Query")) -> ()
                        n902 = local write "Update"(FALSE ("Query")) -> ()
                        n903 = local write "Delete"(FALSE ("Query")) -> ()
                        n904 = local write "Save"(FALSE ("Query")) -> ()
                      }
                    }
                  }
                  frame #2 {
                    w1088 = u16 0 items=["", "Common", "H3C psw 10G", "H3C psw 28G"] ("CmdType")
                    # "清空数组"
                    n905 = control-ref of="Report Templete Path:"() -> (w1092:refnum<vi>)
                    n906 = control-ref of="Data Points"() -> (w1091:refnum<vi>)
                    n907 = control-ref of="Spec _Data"() -> (w1090:refnum<vi>)
                    n908 = local write "CmdType"(w1088) -> ()
                    n909 = local read "bool"() -> (w1089:refnum<vi>[])
                    n910 = local read "number"() -> (w1093:refnum<vi>[])
                    n911 = local read "string"() -> (w1096:refnum<vi>[])
                    n912 = local read "chart"() -> (w1094:refnum<vi>[])
                    n913 = local read "list"() -> (w1095:refnum<vi>[])
                    n914 = call "_wmg_initAllCtrls.vi"("chart"=w1094, "number"=w1093, "list"=w1095, "string"=w1096, "bool"=w1089, "Spec _Data"=w1090, "Data Points"=w1091, "Report Templete Path:"=w1092) -> ()
                    n915 = property on="Update" class="Bool (严格)"("DisabledEnum"=T4."Disabled and Grayed Out" ("禁用")) -> ()  [unwired: 2 in, 2 out]
                    n916 = property on="Delete" class="Bool (严格)"("DisabledEnum"=T4."Disabled and Grayed Out" ("禁用")) -> ()  [unwired: 2 in, 2 out]
                    n917 = property on="Luxshare_P/N:" class="Str"("DisabledEnum"=T4."Disabled and Grayed Out" ("禁用")) -> ()  [unwired: 2 in, 2 out]
                    n918 = local write "Query"(FALSE ("Query")) -> ()
                    n919 = local write "Update"(FALSE ("Query")) -> ()
                    n920 = local write "Delete"(FALSE ("Query")) -> ()
                    n921 = local write "Save"(FALSE ("Query")) -> ()
                  }
                }
              }
              frame 10 {
                n922 = stacked-sequence {
                  frame #0 {
                    n923 = local read "Local"() -> (w1104:bool)
                    n924 = case shown="假" w1104 {
                      frame False {
                        n925 = local read "Luxshare_P/N:"() -> (w1112:string)
                        n926 = property on="System_Mode" class="Ring (严格)"() -> ("RingText.Text"=w1108:string)  [unwired: 2 in, 2 out]
                        n927 = call "_wmg_HardModetoHardModewhereConnect.vi"("Input"=w1108) -> ("Output"=w1106:string)
                        n928 = call "_wmg_PNtoPNwhereConnect.vi"("Input"=w1112) -> ("Output"=w1107:string)
                        n929 = Concatenate Strings(w1107, w1106) -> (w1105:string)
                        n930 = call "sql-delete.vi"("操作模式"=T8."删除数据", "限定条件"=w1105) -> ("错误类型"=w1109:string, "status"=w1110:bool)  [unwired: 16 in]
                        n931 = case shown="假" w1110 {
                          tunnel: ["数据删除成功！" ("消息") w1115] -> w1111
                          tunnel: w1109 -> [_ w1115]
                          frame False {
                          }
                          frame True {
                          }
                        }
                        n932 = One Button Dialog(message=w1111) -> ()  [unwired: 1 in, 1 out]
                      }
                      frame True {
                        n933 = local read "Luxshare_P/N:"() -> (w1121:string)
                        n934 = call <vilib>:"Application Directory.vi"() -> ("Application Directory"=w1125:path)
                        n935 = Concatenate Strings("Database\\" ("字符串"), w1121, ".hpj" ("字符串")) -> (w1124:string)
                        n936 = Build Path(base path=w1125, name or relative path=w1124) -> (appended path=w1120:path)
                        n937 = Delete(path (use dialog)=w1120) -> (error out=w1116:errorcluster)  [unwired: 4 in, 2 out]
                        n938 = Unbundle(w1116) -> ("status"=w1119:bool, "source"=w1117:string)  [unwired: 1 out]
                        n939 = case shown="假" w1119 {
                          tunnel: ["文件删除成功！" ("消息") w1127] -> w1118
                          tunnel: w1117 -> [_ w1127]
                          frame False {
                          }
                          frame True {
                          }
                        }
                        n940 = One Button Dialog(message=w1118) -> ()  [unwired: 1 in, 1 out]
                      }
                    }
                  }
                  frame #1 {
                    w1128 = u16 0 items=["", "Common", "H3C psw 10G", "H3C psw 28G"] ("CmdType")
                    # "清空数组"
                    n941 = control-ref of="Report Templete Path:"() -> (w1139:refnum<vi>)
                    n942 = control-ref of="Data Points"() -> (w1138:refnum<vi>)
                    n943 = control-ref of="Spec _Data"() -> (w1137:refnum<vi>)
                    n944 = local write "CmdType"(w1128) -> ()
                    n945 = local read "bool"() -> (w1129:refnum<vi>[])
                    n946 = local read "number"() -> (w1140:refnum<vi>[])
                    n947 = local read "string"() -> (w1143:refnum<vi>[])
                    n948 = local read "chart"() -> (w1141:refnum<vi>[])
                    n949 = local read "list"() -> (w1142:refnum<vi>[])
                    n950 = call "_wmg_initAllCtrls.vi"("chart"=w1141, "number"=w1140, "list"=w1142, "string"=w1143, "bool"=w1129, "Spec _Data"=w1137, "Data Points"=w1138, "Report Templete Path:"=w1139) -> ()
                    n951 = property on="Update" class="Bool (严格)"("DisabledEnum"=T4."Disabled and Grayed Out" ("禁用")) -> ()  [unwired: 2 in, 2 out]
                    n952 = property on="Delete" class="Bool (严格)"("DisabledEnum"=T4."Disabled and Grayed Out" ("禁用")) -> ()  [unwired: 2 in, 2 out]
                    n953 = property on="Luxshare_P/N:" class="Str"("DisabledEnum"=T4."Disabled and Grayed Out" ("禁用")) -> ()  [unwired: 2 in, 2 out]
                    n954 = local write "Query"(FALSE ("Query")) -> ()
                    n955 = local write "Update"(FALSE ("Query")) -> ()
                    n956 = local write "Delete"(FALSE ("Query")) -> ()
                    n957 = local write "Save"(FALSE ("Query")) -> ()
                  }
                }
              }
              frame 1 {
                n958 = stacked-sequence {
                  frame #0 {
                    w1155 = "@"
                    w1156 = "\r\n"
                    w1166 = "%s" ("格式字符串")
                    n959 = local read "Impedance Spec:"() -> (w1168:string[][])
                    n960 = local read "2X Thru String"() -> (w1152:string)
                    n961 = property on="Delay(ns)" class="DigNum (严格)"() -> ("NumText.Text"=w1150:string)  [unwired: 2 in, 2 out]
                    n962 = property on="Skew max(ps)" class="DigNum (严格)"() -> ("NumText.Text"=w1151:string)  [unwired: 2 in, 2 out]
                    n963 = property on="Start TimeNs" class="DigNum (严格)"() -> ("NumText.Text"=w1149:string)  [unwired: 2 in, 2 out]
                    n964 = property on="StopTimeNs" class="DigNum (严格)"() -> ("NumText.Text"=w1148:string)  [unwired: 2 in, 2 out]
                    n965 = property on="Data Points" class="DigNum (严格)"() -> ("NumText.Text"=w1147:string)  [unwired: 2 in, 2 out]
                    n966 = property on="Filter Risetime(ps)" class="DigNum (严格)"() -> ("NumText.Text"=w1146:string)  [unwired: 2 in, 2 out]
                    n967 = property on="Compensation(ohm)" class="DigNum (严格)"() -> ("NumText.Text"=w1145:string)  [unwired: 2 in, 2 out]
                    n968 = Boolean To (0,1)(Boolean="Impedance Filter") -> (0, 1=w1171:i16)
